vi "meth.CallInternal.vi"(0 "GLue in":refnum<class "class.GLue.lvclass">, 11 "error in":errorcluster) -> (4 "GLue out":refnum<class "class.GLue.lvclass">, 8 "Data out":variant, 13 "Processed?":bool, 15 "error out":errorcluster)   [LabVIEW 2014, in "GLue.lvlib" / "class.GLue.lvclass"]
uses:
  class.GLue.lvclass
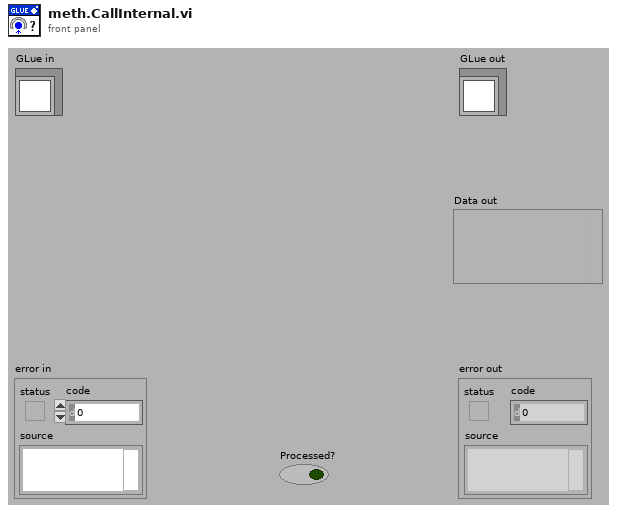
[diagram p1: front panel]
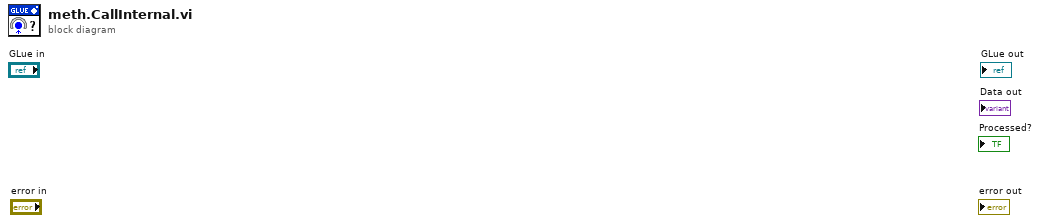
[diagram p0: block diagram]
diagram:
